vi "Get Bytes.vi"(11 "MsgPackMap in":refnum<class "MsgPackMap.lvclass">) -> (2 "Array":u8[](array[numeric]), 3 "MsgPackMap out":refnum<class "MsgPackMap.lvclass">)   [LabVIEW 2020, in "MessagePack.lvlib" / "MsgPackMap.lvclass"]
uses:
  MsgPackMap.lvclass
  MsgPackMap.lvclass/MsgPackMap.ctl
  MsgPack Object Types.ctl
  MessagePack.lvclass
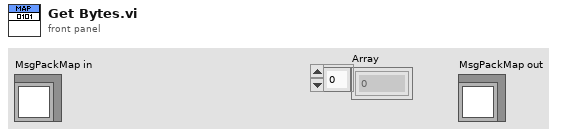
[diagram p1: front panel]
types:
  T1 = typedef "MessagePack.lvlib/MessagePack.lvclass/MsgPack Object Types.ctl" = enum16{"UNSUPPORTED", "POSINT", "NEGINT", "FIXMAP", "FIXARRAY", "FIXSTR", "NIL", "FALSE", "TRUE", "BIN8", "BIN16", "BIN32", "EXT8", "EXT16", "EXT32", "FLOAT32", "FLOAT64", "UINT8", "UINT16", "UINT32", "UINT64", "INT8", "INT16", "INT32", "INT64", "FIXEXT1", "FIXEXT2", "FIXEXT4", "FIXEXT8", "FIXEXT16", "STR8", "STR16", "STR32", "ARRAY16", "ARRAY32", "MAP16", "MAP32"}
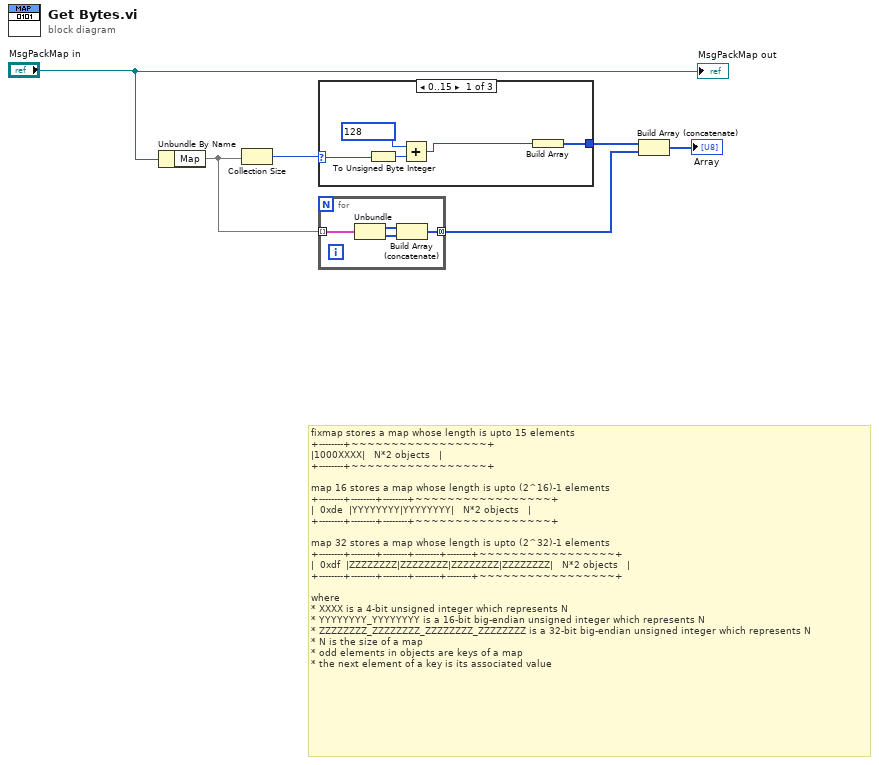
[diagram p0: block diagram]
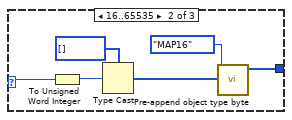
[diagram p2: hidden frame]
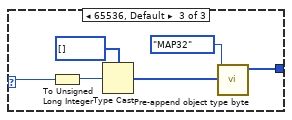
[diagram p3: hidden frame]
diagram:
  # "fixmap stores a map whose length is upto 15 elements\n+--------+~~~~~~~~~~~~~~~~~+\n|1000XXXX|   N*2 objects   |\n+--------+~~~~~~~~~~~~~~~~~+\n\nmap 16 stores a map whose length is upto (2^16)-1 elements\n+--------+--------+--------+~~~~~~~~~~~~~~~~~+\n|  0xde  |YYYYYYYY|YYYYYYYY|   N*2 objects   |\n+--------+--------+--------+~~~~~~~~~~~~~~~~~+\n\nmap 32 stores a map whose length is upto (2^32)-1 elements\n+--------+--------+--------+--------+--------+~~~~~~~~~~~~~~~~~+\n|  0xdf  |ZZZZZZZZ|ZZZZZZZZ|ZZZZZZZZ|ZZZZZZZZ|   N*2 objects   |\n+--------+--------+--------+--------+--------+~~~~~~~~~~~~~~~~~+\n\nwhere\n* XXXX is a 4-bit unsigned integer which represents N\n* YYYYYYYY_YYYYYYYY is a 16-bit big-endian unsigned integer which represents N\n* ZZZZZZZZ_ZZZZZZZZ_ZZZZZZZZ_ZZZZZZZZ is a 32-bit big-endian unsigned integer which represents N\n* N is the size of a map\n* odd elements in objects are keys of a map\n* the next element of a key is its associated value"
  n1 = Unbundle By Name("MsgPackMap in") -> ("Map"=w3:map{u8[], u8[]})
  n2 = Collection Size(1:w3) -> (0:w2:i32)
  n3 = case shown="0..15" w2 {
    selector: w2 -> [w10 w17 w23]
    tunnel: [w8 w13 w19] -> w6
    frame 0..15 {
      n4 = To Unsigned Byte Integer(number=w10) -> (unsigned 8bit integer=w9:u8)
      n5 = Add(x=u8 128 ("y"), y=w9) -> (x+y=w7:u8)
      n6 = Build Array(w7) -> (w8:u8[])
    }
    frame 16..65535 {
      n7 = To Unsigned Word Integer(number=w17) -> (unsigned 16bit integer=w15:u16)
      n8 = Type Cast(type=u8[] [] ("bytes"), x=w15) -> (*(type *) &x=w14:u8[])
      n9 = call "Pre-append object type byte.vi"("bytes in"=w14, "Object type"=MsgPack_Object_Types."MAP16") -> ("encoded bytes"=w13:u8[])  [unwired: 8 in, 1 out]
    }
    frame 65536, Default {
      n10 = To Unsigned Long Integer(number=w23) -> (unsigned 32bit integer=w21:u32)
      n11 = Type Cast(type=u8[] [] ("bytes"), x=w21) -> (*(type *) &x=w20:u8[])
      n12 = call "Pre-append object type byte.vi"("bytes in"=w20, "Object type"=MsgPack_Object_Types."MAP32") -> ("encoded bytes"=w19:u8[])  [unwired: 8 in, 1 out]
    }
  }
  n13 = for {
    tunnel: w3 -> [w27] mode=indexing
    tunnel: [w24] -> w1 mode=concatenating
    n14 = Unbundle(w27) -> ("Key"=w26:u8[], "Value"=w25:u8[])
    n15 = Build Array (concatenate)(w26, w25) -> (w24:u8[])
  }
  n16 = Build Array (concatenate)(w6, w1) -> (→"Array":u8[])
  "MsgPackMap out" <- "MsgPackMap in"
